vi "NavX.vi"(8 "error in":errorcluster) -> ()   [LabVIEW 2015]
uses:
  Z-Old Code/navx-mxp/labview/navX-MXP Library/COMMON/TypeDefs/Value TypeDefs/navX Interface Protocol.ctl
  <vilib>/Rock Robotics/SystemInterfaces/i2clib/i2c_bus.ctl
  LED Lights/LED Lights Global.vi
  NavX Global.vi
  <vilib>/Rock Robotics/Network Tables/NT Write Number.vi
  Z-Old Code/navx-mxp/labview/navX-MXP Library/navX-MXP IMU.lvlib
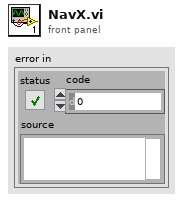
[diagram p1: front panel]
types:
  T1 = typedef "i2c_bus.ctl" = enum16{"I2C On-Board", "I2C MXP", "Invalid"}
  T2 = typedef "navX-MXP IMU.lvlib/navX Interface Protocol.ctl" = enum16{"SPI", "I2C", "SERIAL"}
  T3 = typedef "NavX Light Global Type Def.ctl" = cluster{"NavX Error":errorcluster, "Initialized":bool}
  T4 = typedef "navX-MXP IMU.lvlib/navX Device TypeDef.ctl" = cluster{"navX Interface Protocol":T2, "navX Interface Protocol TypeDefs":cluster{"SPIDevRef":T5, "I2CDevRef":T7}, "navX System Information":cluster{"Board Information":T8, "Status":T11, "Offsets":T15, "LastSampleTimestamp":dbl, "LastSampleValid":bool}, "navX Common Information":cluster{"Update Rate (4Hz-60Hz)":T16, "refnum name":string, "error":errorcluster, "LastSampleFPGATimestamp":dbl}}
  T5 = typedef "WPI_SPIDevRef.ctl" = cluster{"DevStatus":errorcluster, "Handle":i32, "SPI Bus":T6}
  T6 = typedef "spi_bus.ctl" = enum16{"SPI On-Board, CS0", "SPI On-Board, CS1", "SPI On-Board, CS2", "SPI On-Board, CS3", "SPI MXP", "Invalid"}
  T7 = typedef "WPI_I2CDevRef.ctl" = cluster{"DevStatus":errorcluster, "Device Address":u8, "Handle":i32, "I2C Bus":T1}
  T8 = typedef "navX-MXP IMU.lvlib/navX Board Information.ctl" = cluster{"WhoAmI (50 | 0x32)":u8, "Board Revision":u8, "Firmware Major Version":u8, "Firmware Minor Version":u8, "NAVX_BOARD_CAPABILITY":T9, "NAVX_BOARD_YAW_AXIS":T10}
  T9 = typedef "navX-MXP IMU.lvlib/navX NAVX_BOARD_CAPABILITY.ctl" = cluster{"OMNIMOUNT":bool, "YAW_RESET":bool, "VEL_AND_DISP":bool}
  T10 = typedef "navX-MXP IMU.lvlib/navX NAVX_BOARD_YAW_AXIS.ctl" = cluster{"BOARD_YAW_AXIS_UP":bool, "BOARD_YAW_AXIS":u8}
  T11 = typedef "navX-MXP IMU.lvlib/navX Status Data.ctl" = cluster{"Update Rate Hz":u8, "Accelerometer Full-Scale Range":u8, "Gyro Full-Scale Range":u16, "NAVX_OP_STATUS":T12, "NAVX_CAL_STATUS":T13, "NAVX_SELFTEST_STATUS":u8, "NAVX_SENSOR_STATUS":T14}
  T12 = typedef "navX-MXP IMU.lvlib/navX NAVX_OP_STATUS.ctl" = u8
  T13 = typedef "navX-MXP IMU.lvlib/navX NAVX_CAL_STATUS.ctl" = u8
  T14 = typedef "navX-MXP IMU.lvlib/navX NAVX_SENSOR_STATUS.ctl" = cluster{"MOVING":bool, "YAW_STABLE":bool, "MAG_DISTURBANCE":bool, "ALTITUDE_VALID":bool, "SEALEVEL_PRESS_SET":bool, "FUSED_HEADING_VALID":bool}
  T15 = typedef "navX-MXP IMU.lvlib/navX Offsets Data.ctl" = cluster{"Yaw":dbl, "Quat W":dbl, "Quat X":dbl, "Quat Y":dbl, "Quat Z":dbl}
  T16 = typedef "navX-MXP IMU.lvlib/navX Update Rate.ctl" = u8
  T17 = typedef "navX-MXP IMU.lvlib/navX YPRH Data.ctl" = cluster{"Yaw":dbl, "Pitch":dbl, "Roll":dbl, "Heading":dbl}
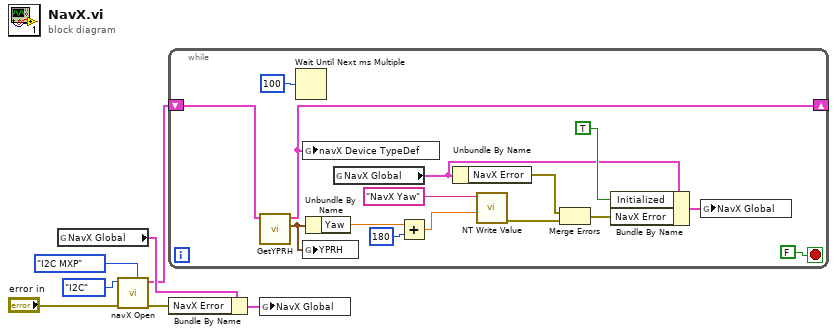
[diagram p0: block diagram]
diagram:
  n1 = global read "LED Lights Global.vi" "NavX Global"() -> (w4:T3)
  n2 = call "navX Open.vi"("I2C Bus"=i2c_bus."I2C MXP", "error in"="error in", "navX Interface Protocol"=navX_Interface_Protocol."I2C") -> ("error out"=w2:errorcluster, "navX Device TypeDef"=w1:T4)  [unwired: 6 in, 1 out]
  n3 = while {
    shift-right: [w8] -> _
    shift-left: w1 -> [w10]
    stop <- FALSE stop-if-true
    n4 = call "GetYPRH.vi"("navX Device TypeDef"=w10) -> ("YPRH"=w9:T17, "navX Device TypeDef"=w8:T4)  [unwired: 8 in, 1 out]
    n5 = Wait Until Next ms Multiple(millisecond multiple=u32 100) -> ()  [unwired: 1 out]
    n6 = global write "NavX Global.vi" "navX Device TypeDef"(w8) -> ()
    n7 = global write "NavX Global.vi" "YPRH"(w9) -> ()
    n8 = Unbundle By Name(w9) -> ("Yaw"=w19:dbl)
    n9 = global read "LED Lights Global.vi" "NavX Global"() -> (w13:T3)
    n10 = Add(x=w19, y=180) -> (x+y=w17:dbl)
    n11 = Unbundle By Name(w13) -> ("NavX Error"=w11:errorcluster)
    n12 = call-poly <vilib>:"NT Write Value.vi"("Numeric"=w17, "Name"="NavX Yaw") -> ("error out"=w14:errorcluster)  [unwired: 9 in]
    n13 = Merge Errors(w11, w14) -> (w15:errorcluster)
    n14 = Bundle By Name(cluster=w13, "Initialized"=TRUE, "NavX Error"=w15) -> (w12:T3)
    n15 = global write "LED Lights Global.vi" "NavX Global"(w12) -> ()
  }
  n16 = Bundle By Name(cluster=w4, "NavX Error"=w2) -> (w3:T3)
  n17 = global write "LED Lights Global.vi" "NavX Global"(w3) -> ()
